vi "DatabaseHand_Element_Get(path).vi"(7 "nd queue":bool, 8 "error in (no error)":errorcluster, 9 "default value":path, 10 "name":string, 11 "Database RefNum in":T1) -> (0 "error out":errorcluster, 1 "type":string, 2 "value":path, 3 "Database RefNum out":T1, 4 "permissions":string="RW", 5 "group":string, 6 "unit":string)   [LabVIEW 2016]
doc: "This VI finds the RefNum of an existing object with the input Name or creates a new object if the Name is not found or Name is unwired or an empty string.\nCopyright 2001 VI Engineering, Inc."
uses:
  DatabaseHand_RefNum.ctl
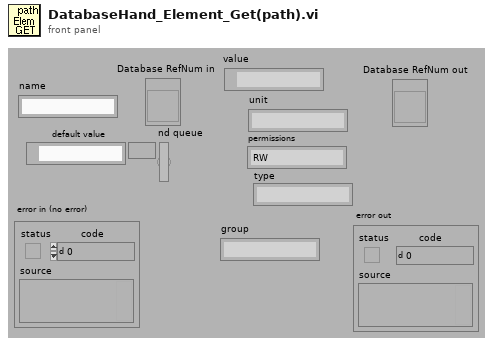
[diagram p1: front panel]
types:
  T1 = typedef "DatabaseHand_RefNum.ctl" = refnum<vi>
  T2 = typedef "DatabaseHand_Element.ctl" = cluster{"name":string, "Database":T3[]}
  T3 = typedef "DatabaseHan_DatabaseElement.ctl" = cluster{"name":string, "value":string, "type":string, "unit":string, "permissions":string, "enqueued":bool, "group":string}
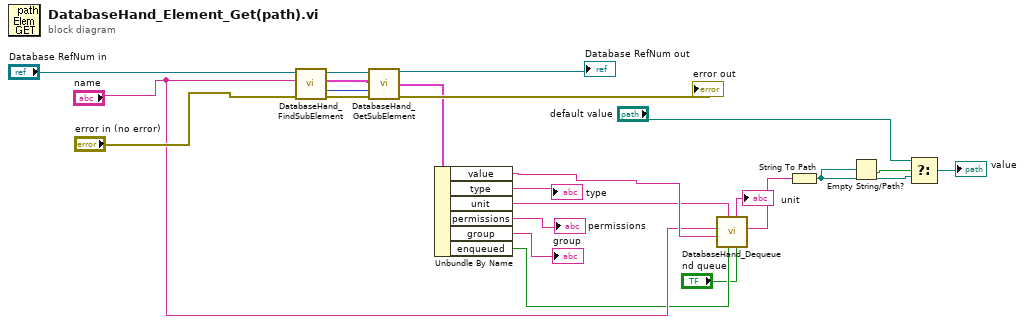
[diagram p0: block diagram]
diagram:
  n1 = call "DatabaseHand_FindSubElement.vi"("error in (no error)"="error in (no error)", "name"="name", "Database RefNum in"="Database RefNum in") -> ("error out"=w19:errorcluster, "index"=w16:i32, "Database"=w20:T2, "Database RefNum out"=w21:T1)  [unwired: 5 out]
  n2 = call "DatabaseHand_GetSubElement.vi"("Database RefNum in"=w21, "Object Data In"=w20, "Index"=w16, "error in (no error)"=w19) -> ("Database RefNum out"=→"Database RefNum out":T1, "Element found"=w15:T3, "error out"=→"error out":errorcluster)  [unwired: 9 out]
  n3 = Unbundle By Name(w15) -> ("value"=w7:string, "type"=→"type":string, "unit"=w2:string, "permissions"=→"permissions":string, "group"=→"group":string, "enqueued"=w5:bool)
  n4 = call "DatabaseHand_Dequeue.vi"("non-destructive queue"="nd queue", "queue?"=w5, "unit in"=w2, "value in"=w7, "name"="name") -> ("value out"=w4:string, "unit out"=→"unit":string)  [unwired: 5 out]
  n5 = String To Path(string=w4) -> (path=w10:path)
  n6 = Empty String/Path?(string/path=w10) -> (empty?=w12:bool)
  n7 = Select(t="default value", s=w12, f=w10) -> (s? t:f=→"value":path)
